vi "Autonomous Two Ball.vi"() -> ()   [LabVIEW 2013]
uses:
  Auto Two Ball States.ctl
  Autonomous Actuator References.ctl
  <vilib>/Rock Robotics/WPI/Solenoid/WPI_SolenoidDevRef.ctl
  <vilib>/Rock Robotics/SystemInterfaces/Typedef/FPGA_TypedefSolenoidModule.ctl
  <vilib>/Rock Robotics/WPI/Solenoid/WPI_SolenoidChannel.ctl
  <vilib>/Rock Robotics/WPI/MotorControl/WPI_MotorControlDeviceRef.ctl
  <vilib>/Rock Robotics/SystemInterfaces/Typedef/FPGA_TypedefDigitalModule.ctl
  <vilib>/Rock Robotics/SystemInterfaces/DIO/FPGA_DIOPWMChannel.ctl
  <vilib>/Rock Robotics/WPI/PWM/WPI_PWMDeadband.ctl
  <vilib>/Rock Robotics/WPI/CAN/Jaguar/SubVIs/WPI_CANJaguar_ControlMode.ctl
  <vilib>/Rock Robotics/WPI/PWM/WPI_PWMTransform_ConPane.ctl
  <vilib>/Rock Robotics/WPI/RobotDrive/WPI_RobotDriveDevRef.ctl
  Autonomous Sensor References.ctl
  <vilib>/Rock Robotics/WPI/DigitalInput/WPI_DigitalInputDevRef.ctl
  <vilib>/Rock Robotics/SystemInterfaces/DIO/FPGA_DIOChannel.ctl
  Autonomous Actuator Values.ctl
  <vilib>/Rock Robotics/WPI/Solenoid/WPI_SolenoidValue.ctl
  <vilib>/Rock Robotics/WPI/RobotDrive/WPI_RobotDriveGetSetRefNum.vi
panel:
  out "Loop Time":u32(graph)
  out "State":i16(graph)
  out "Current State":T1=enum."Grab Second Ball Wait"
  out "Reset":i16(graph)
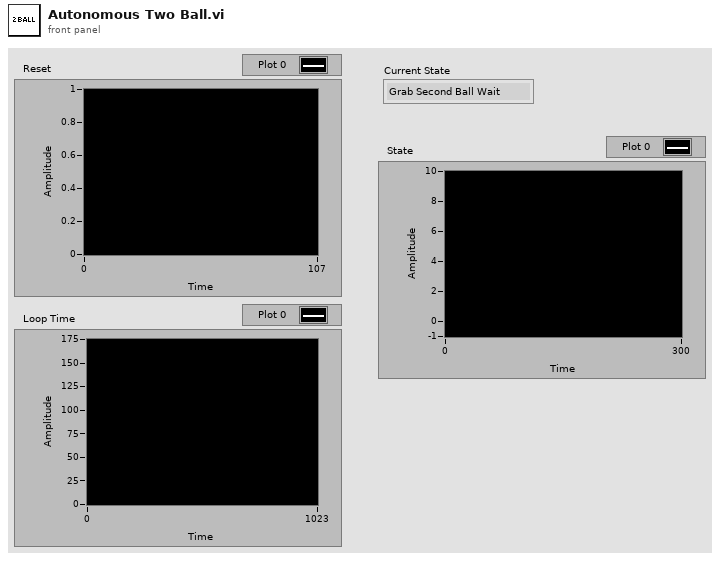
[diagram p1: front panel]
types:
  T1 = typedef "Auto Two Ball States.ctl" = enum16{"Initial Retract", "Initial Retract Wait", "First Shot: Wait for ball", "First Shot: Shoot", "Second Shot: Wait for Arm", "Grab Second Ball", "Grab Second Ball Wait", "Second Shot: Wait for ball", "Second Shot: Shoot", "Drive Forward", "Finish"}
  T2 = typedef "Autonomous Sensor References.ctl" = cluster{"Arm Forward":T3, "Arm Back":T3, "Ball Present":T3, "Shooter":T3}
  T3 = typedef "WPI_DigitalInputDevRef.ctl" = cluster{"DevStatus":errorcluster, "DIO Channel":T4, "Digital Module":T5}
  T4 = typedef "FPGA_DIOChannel.ctl" = enum8{"DIO 1", "DIO 2", "DIO 3", "DIO 4", "DIO 5", "DIO 6", "DIO 7", "DIO 8", "DIO 9", "DIO 10", "DIO 11", "DIO 12", "DIO 13", "DIO 14", "Invalid"}
  T5 = typedef "FPGA_TypedefDigitalModule.ctl" = enum16{"Digital Module 1", "Digital Module 2"}
  T6 = typedef "Autonomous Actuator References.ctl" = cluster{"Arm Fingers":T7, "Arm":T7, "Roller":T10, "Shooter":T10, "Drive":T16, "Gearing":T7}
  T7 = typedef "WPI_SolenoidDevRef.ctl" = cluster{"DevStatus":errorcluster, "Solenoid Module":T8, "Forward Solenoid Channel":T9, "Reverse Solenoid Channel":T9}
  T8 = typedef "FPGA_TypedefSolenoidModule.ctl" = enum16{"Solenoid Module 1", "Solenoid Module 2"}
  T9 = typedef "WPI_SolenoidChannel.ctl" = enum8{"Solenoid 1", "Solenoid 2", "Solenoid 3", "Solenoid 4", "Solenoid 5", "Solenoid 6", "Solenoid 7", "Solenoid 8", "Invalid"}
  T10 = typedef "WPI_MotorControlDeviceRef.ctl" = cluster{"DeviceStatus":errorcluster, "Type":enum16{"PWM", "CAN"}, "PWM":cluster{"Digital Module":T5, "PWM Channel":T11, "DeadBand":T12}, "CAN":cluster{"Device Number":u8, "Control Mode":T13, "Semaphore":T14, "Max Vout":dbl}, "Invert":bool, "TransformRef":T15, "InvTransformRef":T15}
  T11 = typedef "FPGA_DIOPWMChannel.ctl" = enum8{"PWM 1", "PWM 2", "PWM 3", "PWM 4", "PWM 5", "PWM 6", "PWM 7", "PWM 8", "PWM 9", "PWM 10", "Invalid"}
  T12 = typedef "WPI_PWMDeadband.ctl" = cluster{"Name":string, "maxPositivePwm":i32, "minPositivePwm":i32, "centerPwm":i32, "maxNegativePwm":i32, "minNegativePwm":i32, "angularRange":u16}
  T13 = typedef "WPI_CANJaguar_ControlMode.ctl" = enum8{"Percent VBus", "Current", "Speed", "Position", "Voltage"}
  T14 = typedef "Semaphore RefNum" = refnum<k1>
  T15 = typedef "WPI_PWMTransform_ConPane.ctl" = refnum<vi>
  T16 = typedef "WPI_RobotDriveDevRef.ctl" = cluster{"DevStatus":errorcluster, "Motors[]":T10[], "Square Inputs":bool, "Max Output":dbl, "Isochronous":bool}
  T17 = typedef "WPI_SolenoidValue.ctl" = enum16{"Off", "On", "Forward", "Reverse"}
  T18 = typedef "Autonomous Actuator Values.ctl" = cluster{"Arm Fingers":T17, "Arm":T17, "Roller":dbl, "Shooter":dbl, "X":dbl, "Y":dbl, "Gearing":T17}
  T19 = typedef "Autonomous Sensor Values.ctl" = cluster{"Arm Forward":bool, "Arm Back":bool, "Ball Present":bool, "Shooter":bool}
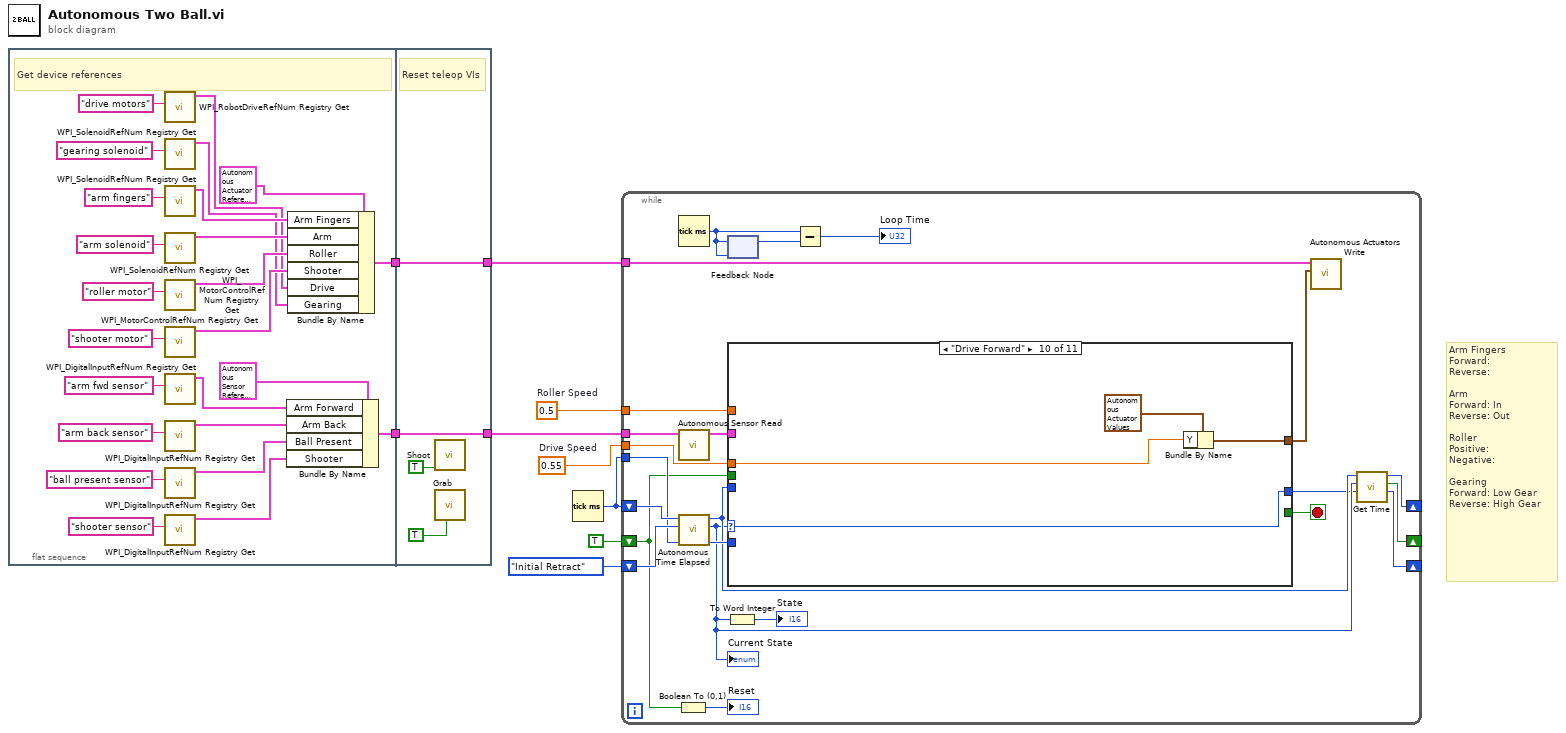
[diagram p0: block diagram]
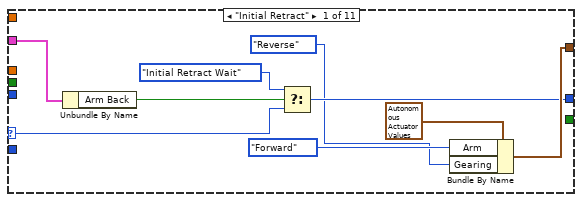
[diagram p2: hidden frame]
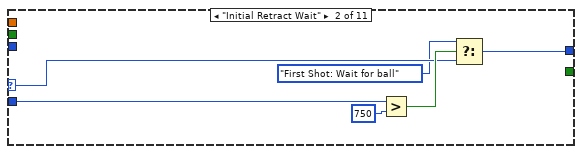
[diagram p3: hidden frame]
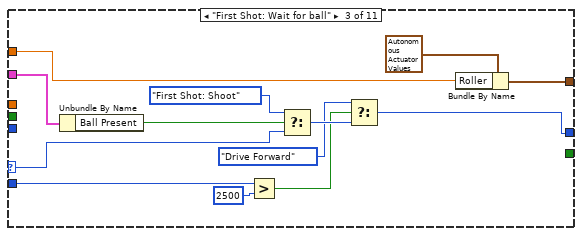
[diagram p4: hidden frame]
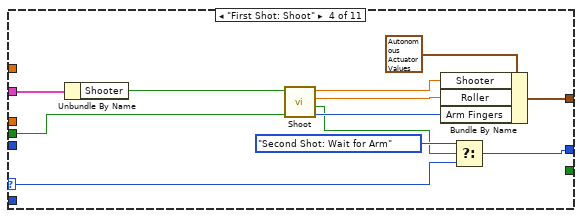
[diagram p5: hidden frame]
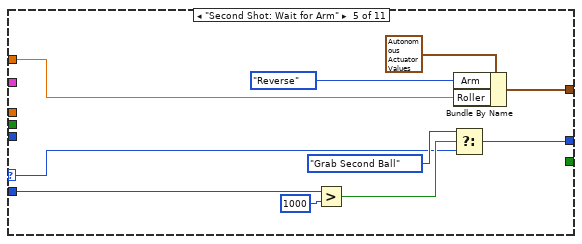
[diagram p6: hidden frame]
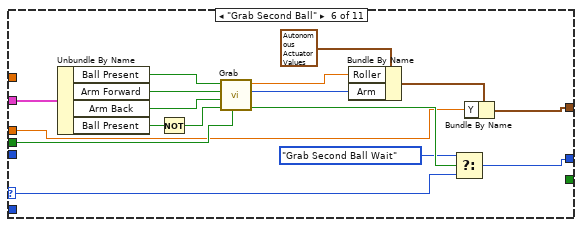
[diagram p7: hidden frame]
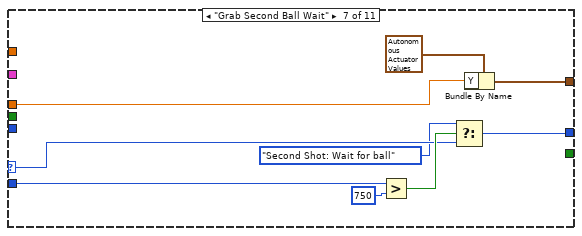
[diagram p8: hidden frame]
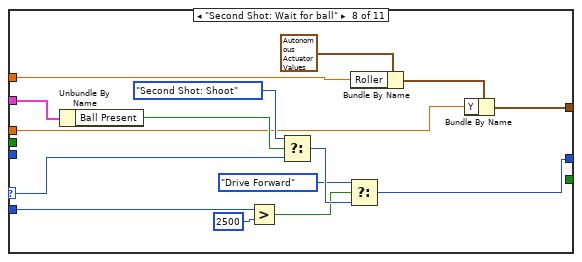
[diagram p9: hidden frame]
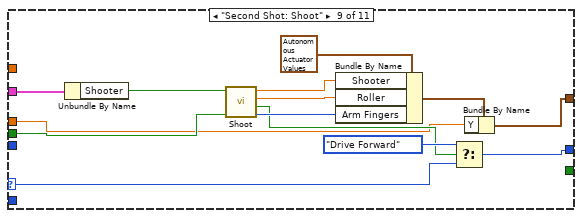
[diagram p10: hidden frame]
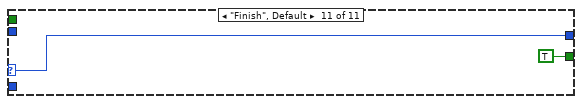
[diagram p11: hidden frame]
diagram:
  w3 = 0.5  # Roller Speed
  w4 = 0.55  # Drive Speed
  # "Arm Fingers\nForward:\nReverse:\n\nArm\nForward: In\nReverse: Out\n\nRoller\nPositive:\nNegative:\n\nGearing\nForward: Low Gear\nReverse: High Gear"
  n1 = flat-sequence {
    tunnel: [w18] -> w2
    tunnel: [w12] -> w1
    tunnel: [w36] -> w6
    tunnel: [w37] -> w7
    tunnel: w2 -> [w37]
    tunnel: w1 -> [w36]
    frame #0 {
      # "Get device references"
      n2 = call <vilib>:"WPI_RobotDriveRefNum Registry Get.vi"("refnum name"="drive motors") -> ("RobotDriveDevRef"=w20:T16)  [unwired: 9 in, 1 out]
      n3 = call <vilib>:"WPI_SolenoidRefNum Registry Get.vi"("refnum name"="gearing solenoid") -> ("SolenoidDevRef"=w10:T7)  [unwired: 9 in, 1 out]
      n4 = call <vilib>:"WPI_SolenoidRefNum Registry Get.vi"("refnum name"="arm fingers") -> ("SolenoidDevRef"=w24:T7)  [unwired: 9 in, 1 out]
      n5 = call <vilib>:"WPI_SolenoidRefNum Registry Get.vi"("refnum name"="arm solenoid") -> ("SolenoidDevRef"=w23:T7)  [unwired: 9 in, 1 out]
      n6 = call <vilib>:"WPI_MotorControlRefNum Registry Get.vi"("refnum name"="roller motor") -> ("MotorControlDevRef"=w22:T10)  [unwired: 9 in, 1 out]
      n7 = call <vilib>:"WPI_MotorControlRefNum Registry Get.vi"("refnum name"="shooter motor") -> ("MotorControlDevRef"=w21:T10)  [unwired: 9 in, 1 out]
      n8 = call <vilib>:"WPI_DigitalInputRefNum Registry Get.vi"("refnum name"="arm fwd sensor") -> ("DigitalInputDevRef"=w16:T3)  [unwired: 9 in, 1 out]
      n9 = call <vilib>:"WPI_DigitalInputRefNum Registry Get.vi"("refnum name"="arm back sensor") -> ("DigitalInputDevRef"=w14:T3)  [unwired: 9 in, 1 out]
      n10 = call <vilib>:"WPI_DigitalInputRefNum Registry Get.vi"("refnum name"="ball present sensor") -> ("DigitalInputDevRef"=w15:T3)  [unwired: 9 in, 1 out]
      n11 = call <vilib>:"WPI_DigitalInputRefNum Registry Get.vi"("refnum name"="shooter sensor") -> ("DigitalInputDevRef"=w13:T3)  [unwired: 9 in, 1 out]
      n12 = Bundle By Name(cluster=T2 {"Arm Forward"={"DevStatus"={"status"=FALSE, "code"=0, "source"=""}, "DIO Channel"=enum."DIO 1", "Digital Module"=enum."Digital Module 1"}, "Arm Back"={"DevStatus"={"status"=FALSE, "code"=0, "source"=""}, "DIO Channel"=enum."DIO 1", "Digital Module"=enum."Digital Module 1"}, "Ball Present"={"DevStatus"={"status"=FALSE, "code"=0, "source"=""}, "DIO Channel"=enum."DIO 1", "Digital Module"=enum."Digital Module 1"}, "Shooter"={"DevStatus"={"status"=FALSE, "code"=0, "source"=""}, "DIO Channel"=enum."DIO 1", "Digital Module"=enum."Digital Module 1"}} ("output cluster"), "Arm Forward"=w16, "Arm Back"=w14, "Ball Present"=w15, "Shooter"=w13) -> (w12:T2)
      n13 = Bundle By Name(cluster=T6 {"Arm Fingers"={"DevStatus"={"status"=FALSE, "code"=0, "source"=""}, "Solenoid Module"=enum."Solenoid Module 1", "Forward Solenoid Channel"=enum."Invalid", "Reverse Solenoid Channel"=enum."Invalid"}, "Arm"={"DevStatus"={"status"=FALSE, "code"=0, "source"=""}, "Solenoid Module"=enum."Solenoid Module 1", "Forward Solenoid Channel"=enum."Invalid", "Reverse Solenoid Channel"=enum."Invalid"}, "Roller"={"DeviceStatus"={"status"=FALSE, "code"=0, "source"=""}, "Type"=enum."PWM", "PWM"={"Digital Module"=enum."Digital Module 1", "PWM Channel"=enum."Invalid", "DeadBand"={"Name"="", "maxPositivePwm"=0, "minPositivePwm"=0, "centerPwm"=0, "maxNegativePwm"=0, "minNegativePwm"=0, "angularRange"=0}}, "CAN"={"Device Number"=0, "Control Mode"=enum."Percent VBus", "Semaphore"=refnum, "Max Vout"=12.0}, "Invert"=FALSE, "TransformRef"=refnum, "InvTransformRef"=refnum}, "Shooter"={"DeviceStatus"={"status"=FALSE, "code"=0, "source"=""}, "Type"=enum."PWM", "PWM"={"Digital Module"=enum."Digital Module 1", "PWM Channel"=enum."Invalid", "DeadBand"={"Name"="", "maxPositivePwm"=0, "minPositivePwm"=0, "centerPwm"=0, "maxNegativePwm"=0, "minNegativePwm"=0, "angularRange"=0}}, "CAN"={"Device Number"=0, "Control Mode"=enum."Percent VBus", "Semaphore"=refnum, "Max Vout"=12.0}, "Invert"=FALSE, "TransformRef"=refnum, "InvTransformRef"=refnum}, "Drive"={"DevStatus"={"status"=FALSE, "code"=0, "source"=""}, "Motors[]"=[], "Square Inputs"=FALSE, "Max Output"=1.0, "Isochronous"=FALSE}, "Gearing"={"DevStatus"={"status"=FALSE, "code"=0, "source"=""}, "Solenoid Module"=enum."Solenoid Module 1", "Forward Solenoid Channel"=enum."Solenoid 1", "Reverse Solenoid Channel"=enum."Solenoid 1"}} ("Actuator References"), "Arm Fingers"=w24, "Arm"=w23, "Roller"=w22, "Shooter"=w21, "Drive"=w20, "Gearing"=w10) -> (w18:T6)
    }
    frame #1 {
      # "Reset teleop VIs"
      n14 = call "Shoot.vi"("Reset"=TRUE) -> ()  [unwired: 7 in, 4 out]
      n15 = call "Grab.vi"("Reset"=TRUE) -> ()  [unwired: 8 in, 3 out]
    }
  }
  n16 = Tick Count (ms)() -> (millisecond timer value=w8:u32)
  n17 = while {
    shift-right: [w44] -> _
    shift-left: Auto_Two_Ball_States."Initial Retract" -> [w50]
    tunnel: w8 -> [w45]
    shift-right: [w48] -> _
    shift-left: w8 -> [w46]
    tunnel: w7 -> [w59]
    tunnel: w6 -> [w57]
    shift-right: [w49] -> _
    shift-left: TRUE -> [w39]
    tunnel: w4 -> [w55]
    tunnel: w3 -> [w54]
    stop <- w60 stop-if-true
    n18 = Boolean To (0,1)(Boolean=w39) -> (0, 1=→"Reset":i16)
    n19 = Tick Count (ms)() -> (millisecond timer value=w52:u32)
    n20 = call "Autonomous Sensor Read.vi"("Sensor References"=w57) -> ("Sensor Values"=w56:T19)  [unwired: 10 in]
    n21 = call "Autonomous Time Elapsed.vi"("Match Start Time"=w45, "State in"=w50, "State Start Time"=w46) -> ("State Time Elapsed"=w47:u32, "State out"=w42:T1, "State Start Time out"=w43:u32)  [unwired: 6 in]
    "Current State" <- w42
    n22 = To Word Integer(number=w42) -> (16bit integer=→"State":i16)
    n23 = feedback-in #1(w52) -> ()
    n24 = feedback #1(w52) -> (w53:u32)
    n25 = case shown="\"Drive Forward\"" w42 {
      selector: w42 -> [w62 w72 w87 w93 w106 w118 w133 w150 w158 w166 w170]
      tunnel: [_ _ _ _ _ _ _ _ _ _ TRUE] -> w60
      tunnel: [w66 w71 w84 w91 w108 w116 w132 w147 w156 w166 w170] -> w41
      tunnel: w43 -> [_ _ _ _ _ _ _ _ _ _ _]
      tunnel: w47 -> [_ w75 w82 _ w105 _ w136 w145 _ _ _]
      tunnel: [w68 _ w77 w97 w103 w125 w130 w139 w153 w168 _] -> w58
      tunnel: w56 -> [w67 _ w88 w100 _ w124 _ w151 w165 _ _]
      tunnel: w39 -> [_ _ _ w89 _ w120 _ _ w163 _ _]
      tunnel: w55 -> [_ _ _ _ _ w111 w129 w138 w152 w167 _]
      tunnel: w54 -> [_ _ w76 _ w101 _ _ w137 _ _ _]
      frame "Initial Retract" {
        n26 = Unbundle By Name(w67) -> ("Arm Back"=w64:bool)
        n27 = Select(t=Auto_Two_Ball_States."Initial Retract Wait" ("f"), s=w64, f=w62) -> (s? t:f=w66:T1)
        n28 = Bundle By Name(cluster=T18 {"Arm Fingers"=enum."Off", "Arm"=enum."Off", "Roller"=0.0, "Shooter"=0.0, "X"=0.0, "Y"=0.0, "Gearing"=enum."Off"} ("Actuator Values"), "Arm"=WPI_SolenoidValue."Forward" ("Arm Fingers"), "Gearing"=WPI_SolenoidValue."Reverse") -> (w68:T18)
      }
      frame "Initial Retract Wait" {
        n29 = Greater?(x=w75, y=u32 750) -> (0:w73:bool)
        n30 = Select(t=Auto_Two_Ball_States."First Shot: Wait for ball", s=w73, f=w72) -> (s? t:f=w71:T1)
      }
      frame "First Shot: Wait for ball" {
        n31 = Unbundle By Name(w88) -> ("Ball Present"=w81:bool)
        n32 = Greater?(x=w82, y=u32 2500) -> (0:w79:bool)
        n33 = Select(t=Auto_Two_Ball_States."First Shot: Shoot", s=w81, f=w87) -> (s? t:f=w85:T1)
        n34 = Select(t=Auto_Two_Ball_States."Drive Forward", s=w79, f=w85) -> (s? t:f=w84:T1)
        n35 = Bundle By Name(cluster=T18 {"Arm Fingers"=enum."Off", "Arm"=enum."Off", "Roller"=0.0, "Shooter"=0.0, "X"=0.0, "Y"=0.0, "Gearing"=enum."Off"} ("Actuator Values"), "Roller"=w76) -> (w77:T18)
      }
      frame "First Shot: Shoot" {
        n36 = Unbundle By Name(w100) -> ("Shooter"=w99:bool)
        n37 = call "Shoot.vi"("Reset"=w89, "Shooter Sensor"=w99) -> ("Arm fingers state"=w94:T17, "Finished?"=w90:bool, "Roller Motor Value"=w95:dbl, "Shooter Motor Value"=w96:dbl)  [unwired: 6 in]
        n38 = Bundle By Name(cluster=T18 {"Arm Fingers"=enum."Off", "Arm"=enum."Off", "Roller"=0.0, "Shooter"=0.0, "X"=0.0, "Y"=0.0, "Gearing"=enum."Off"} ("Actuator Values"), "Shooter"=w96, "Roller"=w95, "Arm Fingers"=w94) -> (w97:T18)
        n39 = Select(t=Auto_Two_Ball_States."Second Shot: Wait for Arm", s=w90, f=w93) -> (s? t:f=w91:T1)
      }
      frame "Second Shot: Wait for Arm" {
        n40 = Greater?(x=w105, y=u32 1000) -> (0:w109:bool)
        n41 = Bundle By Name(cluster=T18 {"Arm Fingers"=enum."Off", "Arm"=enum."Off", "Roller"=0.0, "Shooter"=0.0, "X"=0.0, "Y"=0.0, "Gearing"=enum."Off"} ("Actuator Values"), "Arm"=WPI_SolenoidValue."Reverse", "Roller"=w101) -> (w103:T18)
        n42 = Select(t=Auto_Two_Ball_States."Grab Second Ball", s=w109, f=w106) -> (s? t:f=w108:T1)
      }
      frame "Grab Second Ball" {
        n43 = Unbundle By Name(w124) -> ("Ball Present"=w123:bool, "Arm Forward"=w122:bool, "Arm Back"=w121:bool, "Ball Present"=w113:bool)
        n44 = Not(x=w113) -> (.not. x?=w112:bool)
        n45 = call "Grab.vi"("Reset"=w120, "Button Pressed?"=w112, "Arm Back?"=w121, "Arm Forward?"=w122, "Ball Present?"=w123) -> ("Finished?"=w119:bool, "Arm state"=w114:T17, "Roller Speed"=w115:dbl)  [unwired: 4 in]
        n46 = Bundle By Name(cluster=T18 {"Arm Fingers"=enum."Off", "Arm"=enum."Off", "Roller"=0.0, "Shooter"=0.0, "X"=0.0, "Y"=0.0, "Gearing"=enum."Off"} ("Actuator Values"), "Roller"=w115, "Arm"=w114) -> (w126:T18)
        n47 = Select(t=Auto_Two_Ball_States."Grab Second Ball Wait", s=w119, f=w118) -> (s? t:f=w116:T1)
        n48 = Bundle By Name(cluster=w126, "Y"=w111) -> (w125:T18)
      }
      frame "Grab Second Ball Wait" {
        n49 = Greater?(x=w136, y=u32 750) -> (0:w134:bool)
        n50 = Select(t=Auto_Two_Ball_States."Second Shot: Wait for ball", s=w134, f=w133) -> (s? t:f=w132:T1)
        n51 = Bundle By Name(cluster=T18 {"Arm Fingers"=enum."Off", "Arm"=enum."Off", "Roller"=0.0, "Shooter"=0.0, "X"=0.0, "Y"=0.0, "Gearing"=enum."Off"} ("Actuator Values"), "Y"=w129) -> (w130:T18)
      }
      frame "Second Shot: Wait for ball" {
        n52 = Unbundle By Name(w151) -> ("Ball Present"=w144:bool)
        n53 = Greater?(x=w145, y=u32 2500) -> (0:w142:bool)
        n54 = Select(t=Auto_Two_Ball_States."Second Shot: Shoot", s=w144, f=w150) -> (s? t:f=w148:T1)
        n55 = Select(t=Auto_Two_Ball_States."Drive Forward", s=w142, f=w148) -> (s? t:f=w147:T1)
        n56 = Bundle By Name(cluster=T18 {"Arm Fingers"=enum."Off", "Arm"=enum."Off", "Roller"=0.0, "Shooter"=0.0, "X"=0.0, "Y"=0.0, "Gearing"=enum."Off"} ("Actuator Values"), "Roller"=w137) -> (w140:T18)
        n57 = Bundle By Name(cluster=w140, "Y"=w138) -> (w139:T18)
      }
      frame "Second Shot: Shoot" {
        n58 = Unbundle By Name(w165) -> ("Shooter"=w164:bool)
        n59 = call "Shoot.vi"("Reset"=w163, "Shooter Sensor"=w164) -> ("Arm fingers state"=w159:T17, "Finished?"=w155:bool, "Roller Motor Value"=w160:dbl, "Shooter Motor Value"=w161:dbl)  [unwired: 6 in]
        n60 = Bundle By Name(cluster=T18 {"Arm Fingers"=enum."Off", "Arm"=enum."Off", "Roller"=0.0, "Shooter"=0.0, "X"=0.0, "Y"=0.0, "Gearing"=enum."Off"} ("Actuator Values"), "Shooter"=w161, "Roller"=w160, "Arm Fingers"=w159) -> (w154:T18)
        n61 = Select(t=Auto_Two_Ball_States."Drive Forward", s=w155, f=w158) -> (s? t:f=w156:T1)
        n62 = Bundle By Name(cluster=w154, "Y"=w152) -> (w153:T18)
      }
      frame "Drive Forward" {
        n63 = Bundle By Name(cluster=T18 {"Arm Fingers"=enum."Off", "Arm"=enum."Off", "Roller"=0.0, "Shooter"=0.0, "X"=0.0, "Y"=0.0, "Gearing"=enum."Off"} ("Actuator Values"), "Y"=w167) -> (w168:T18)
      }
      frame "Finish", Default {
      }
    }
    n64 = Subtract(x=w52, y=w53) -> (x-y=→"Loop Time":u32)
    n65 = call "Autonomous Actuators Write.vi"("Actuator Values"=w58, "Actuator References"=w59) -> ()  [unwired: 10 in]
    n66 = call "Get Time.vi"("Next State in"=w41, "Current State"=w42, "State Start Time in"=w43) -> ("Next State out"=w44:T1, "Reset"=w49:bool, "State Start Time out"=w48:u32)  [unwired: 6 in]
  }
